vi "Test Time Constant.vi"(8 "error in (no error)":errorcluster, 11 "SR7270 Drivers in":refnum<class "SR7270 Drivers.lvclass">) -> (0 "error out":errorcluster, 3 "SR7270 Drivers out":refnum<class "SR7270 Drivers.lvclass">)   [LabVIEW 2016, in "SR7270 Drivers.lvlib" / "SR7270 Drivers.lvclass"]
uses:
  SR7270 Drivers.lvclass
  Typedefs/TC-NMODE0--enum.ctl
  Typedefs/NOISEMODE--enum.ctl
  SR7270 Drivers.lvclass/SR7270 Drivers.ctl
  <vilib>/addons/_JKI Toolkits/Caraya/classes/Test/Test.lvclass
  <vilib>/addons/_JKI Toolkits/Caraya/classes/Assert/Assert.lvclass
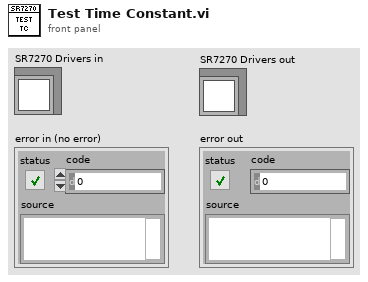
[diagram p1: front panel]
types:
  T1 = typedef "SR7270 Drivers.lvlib/SR7270 Drivers.lvclass/TC-NMODE0--enum.ctl" = enum16{"10 µs", "20 µs", "50 µs", "100 µs", "200 µs", "500 µs", "1 ms", "2 ms", "5 ms", "10 ms", "20 ms", "50 ms", "100 ms", "200 ms", "500 ms", "1 s", "2 s", "5 s", "10 s", "20 s", "50 s", "100 s", "200 s", "500 2", "1 ks", "2 ks", "5 ks", "10 ks", "20 ks", "50 ks", "100 ks"}
  T2 = typedef "SR7270 Drivers.lvlib/SR7270 Drivers.lvclass/NOISEMODE--enum.ctl" = enum16{"OFF", "ON"}
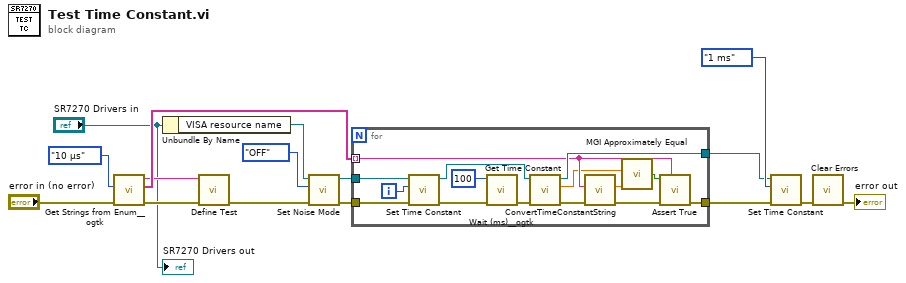
[diagram p0: block diagram]
diagram:
  n1 = call <userlib>:"Get Strings from Enum__ogtk.vi"("error in (no error)"="error in (no error)", "Enum"=TC-NMODE0--enum."10 µs" ("Time Constant-NOISEMODE0")) -> ("error out"=w12:errorcluster, "Enum Strings"=w15:string[], "Enum Name"=w13:string)  [unwired: 6 in, 1 out]
  n2 = Unbundle By Name("SR7270 Drivers in") -> ("VISA resource name"=w2:refnum<visa-resource-name>)
  n3 = call <vilib>:"Define Test.vi"("error in (no error)"=w12, "Label (VI Title)"=w13) -> ("error out"=w8:errorcluster)  [unwired: 9 in]
  n4 = call "Set Noise Mode.vi"("error in (no error)"=w8, "Noise Measurement Mode"=NOISEMODE--enum."OFF", "VISA resource name"=w2) -> ("error out"=w7:errorcluster, "VISA resource name out"=w9:refnum<visa-resource-name>)  [unwired: 7 in]
  n5 = for {
    tunnel: w9 -> [w30]
    tunnel: w7 -> [w25]
    tunnel: [w19] -> w6
    tunnel: [w29] -> w4
    tunnel: w15 -> [w22] mode=indexing
    i -> [w24]
    n6 = call "Set Time Constant.vi"("error in (no error)"=w25, "Time Constant-NOISEMODE0"=w24, "VISA resource name"=w30) -> ("error out"=w26:errorcluster, "VISA resource name out"=w31:refnum<visa-resource-name>)  [unwired: 7 in]
    n7 = call <userlib>:"Wait (ms)__ogtk.vi"("error in (no error)"=w26, "milliseconds to wait"=u32 100) -> ("error out"=w28:errorcluster)  [unwired: 8 in, 1 out]
    n8 = call "Get Time Constant.vi"("error in (no error)"=w28, "VISA resource name"=w31) -> ("error out"=w23:errorcluster, "Time Constant (s)"=w17:dbl, "VISA resource name out"=w29:refnum<visa-resource-name>)  [unwired: 7 in]
    n9 = call "ConvertTimeConstantString.vi"("error in (no error)"=w23, "Time Constant"=w22) -> ("error out"=w21:errorcluster, "Time Constant (s)"=w18:dbl)  [unwired: 8 in]
    n10 = call <userlib>:"MGI Approximately Equal.vi"("Numeric 2"=w18, "Numeric 1"=w17) -> ("approx = ?"=w20:bool)  [unwired: 2 in]
    n11 = call <vilib>:"Assert True.vi"("Label"=w22, "error in (no error)"=w21, "True?"=w20) -> ("error out"=w19:errorcluster)  [unwired: 8 in]
  }
  n12 = call "Set Time Constant.vi"("error in (no error)"=w6, "Time Constant-NOISEMODE0"=TC-NMODE0--enum."1 ms", "VISA resource name"=w4) -> ("error out"=w3:errorcluster)  [unwired: 7 in, 1 out]
  n13 = call <vilib>:"Clear Errors.vi"("error in (no error)"=w3) -> ("error out"=→"error out":errorcluster)  [unwired: 5 in, 1 out]
  "SR7270 Drivers out" <- "SR7270 Drivers in"
